vi "Shutdown--Method.vi"(8 "error in (no error)":errorcluster, 11 "_Thermal Process Controller in":refnum<class "_Thermal Process Controller.lvclass">) -> (0 "error out":errorcluster, 2 "Success?":bool, 3 "_Thermal Process Controller out":refnum<class "_Thermal Process Controller.lvclass">)   [LabVIEW 2024, in "_Thermal Process Controller.lvclass"]
uses:
  _Thermal Process Controller.lvclass
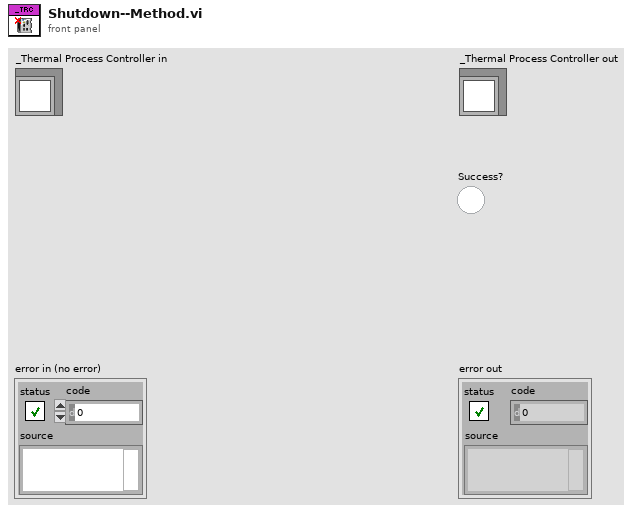
[diagram p1: front panel]
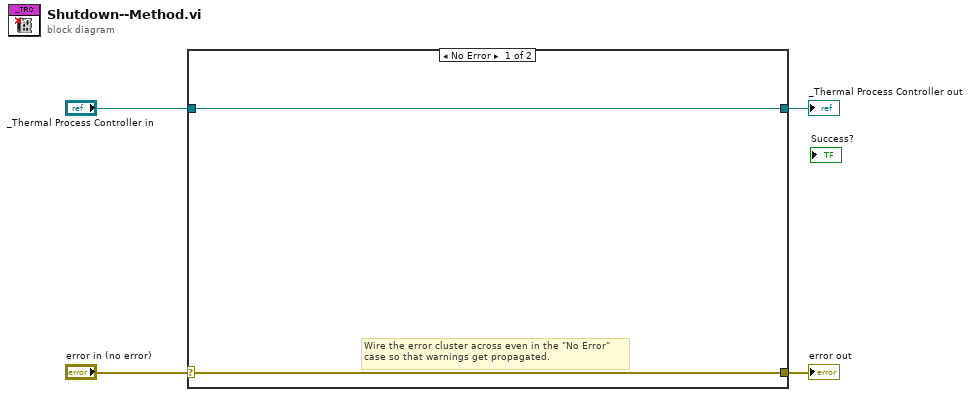
[diagram p0: block diagram]
diagram:
  n1 = case shown="No Error" "error in (no error)" {
    selector: "error in (no error)" -> [w5 w8]
    tunnel: [w5 w8] -> w3
    tunnel: [w6 w7] -> w1
    tunnel: "_Thermal Process Controller in" -> [w6 w7]
    frame No Error {
      # "Wire the error cluster across even in the \"No Error\"\ncase so that warnings get propagated."
    }
    frame Error {
    }
  }
  "error out" <- w3
  "_Thermal Process Controller out" <- w1
